vi "nism.step.p.fxp(modified).vi"(6 "calls per sample":u16, 7 "reset":bool, 8 "minimum pulse":u16, 11 "position setpoint":fxp<+/-,64,32>) -> (0 "position setpoint":fxp<+/-,64,32> format="%.42g", 1 "steps generated":i32, 2 "step":bool, 3 "direction":bool)   [LabVIEW 2015]
doc: "Generates the step and direction pulses necessary to perform stepper motor movement based on position setpoints."
uses:
  <vilib>/rvi/FXPMathLib/FxpDiv/subVIs/nifxpmath_Div_SimConfig.ctl
  <vilib>/rvi/FXPMathLib/FxpDiv/simVIs/DllFxpDivTemp_sub.vi
  <vilib>/rvi/FXPMathLib/FxpAdd/XNode/nifxpmath_Add.xnode
  <vilib>/rvi/FXPMathLib/FxpDiv/XNode/nifxpmath_Div.xnode
  <vilib>/rvi/FXPMathLib/FxpSub/XNode/nifxpmath_Sub.xnode
  <vilib>/Motion/MotorControl/NI_SoftMotion_MotorControlIP.lvlib
  <vilib>/rvi/FXPMathLib/sim/FxpSim.dll
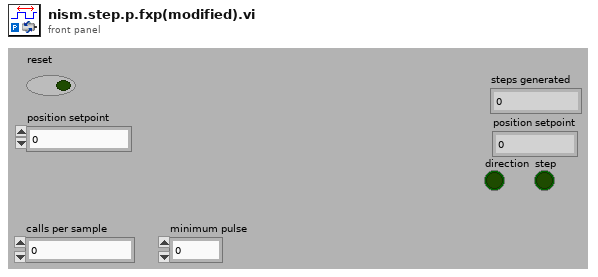
[diagram p1: front panel]
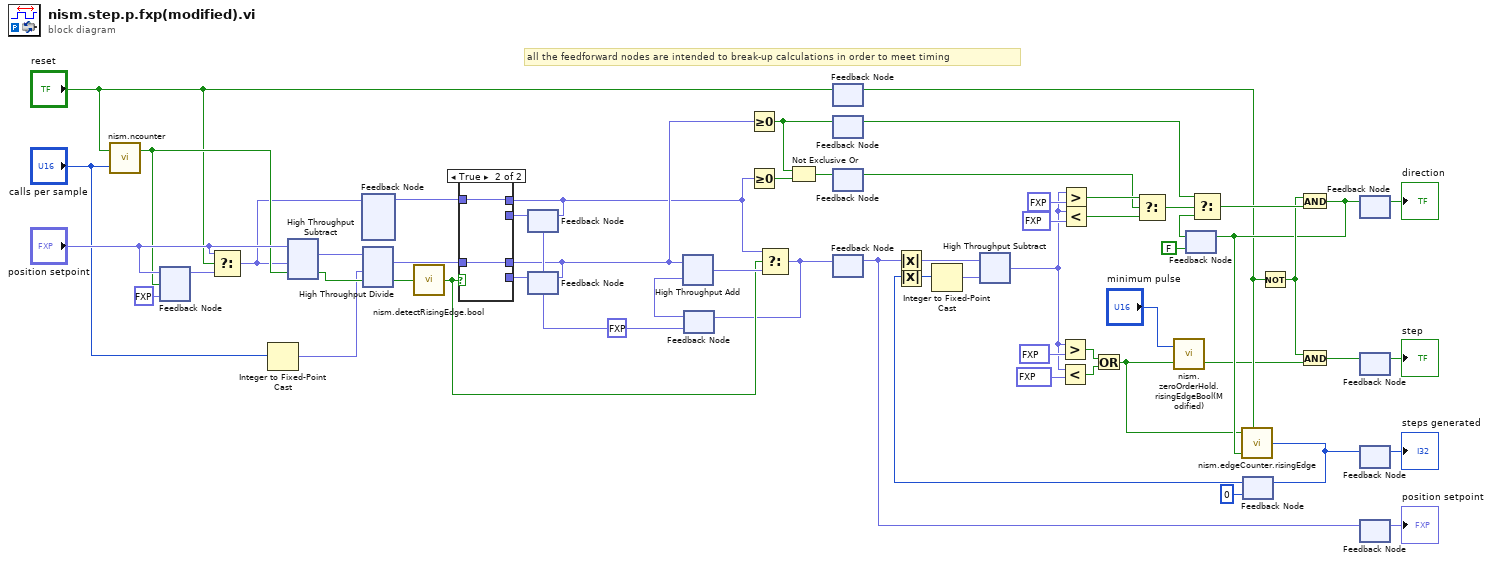
[diagram p0: block diagram]
diagram:
  w50 = fxp<+/-,48,16> 0.0 ("x+y")
  # "all the feedforward nodes are intended to break-up calculations in order to meet timing"
  n1 = call <vilib>:"nism.ncounter.vi"("n"="calls per sample", "reset"="reset") -> ("wrap"=w42:bool)  [unwired: 1 out]
  n2 = feedback #1(fxp<+/-,64,32> 0.0 ("x+y")) -> (w35:fxp<+/-,64,32>)
  n3 = feedback-in #1("position setpoint", w42) -> ()
  n4 = Select(t="position setpoint", s="reset", f=w35) -> (s? t:f=w33:fxp<+/-,64,32>)
  n5 = Integer to Fixed-Point Cast(integer="calls per sample") -> (fixed-point=w23:fxp<+,16,16>)  [unwired: 1 in]
  n6 = xnode ("High Throughput Subtract")("x"="position setpoint", "y"=w33, "input valid"=w42) -> ("x-y"=w28:fxp<+/-,32,16>, "output valid"=w27:bool)  [unwired: 1 in, 1 out]
  n7 = feedback #2() -> (w53:fxp<+/-,64,32>)  [unwired: 1 in]
  n8 = feedback-in #2(w33) -> ()
  n9 = xnode ("High Throughput Divide")("x"=w28, "y"=w23, "input valid"=w27) -> ("x/y"=w25:fxp<+/-,48,16>, "output valid"=w26:bool)  [unwired: 1 in, 1 out]
  n10 = call <vilib>:"nism.detectRisingEdge.bool.vi"("x"=w26) -> ("y"=w19:bool)
  n11 = feedback #3(w50) -> (w52:fxp<+/-,64,32>)
  n12 = feedback #4(w50) -> (w51:fxp<+/-,48,16>)
  n13 = case shown="True" w19 {
    tunnel: w53 -> [_ w62]
    tunnel: w25 -> [_ w61]
    tunnel: [w60 w62] -> w20
    tunnel: [w59 w61] -> w21
    tunnel: w52 -> [w60 _]
    tunnel: w51 -> [w59 _]
    frame False {
    }
    frame True {
    }
  }
  n14 = feedback-in #3(w20) -> ()
  n15 = feedback-in #4(w21) -> ()
  n16 = feedback #5(w50) -> (w55:fxp<+/-,64,32>)
  n17 = xnode ("High Throughput Add")("x"=w21, "y"=w55) -> ("x+y"=w49:fxp<+/-,64,32>)
  n18 = Greater Or Equal To 0?(x=w21) -> (x >= 0?=w9:bool)
  n19 = Greater Or Equal To 0?(x=w20) -> (x >= 0?=w29:bool)
  n20 = Select(t=w20, s=w19, f=w49) -> (s? t:f=w12:fxp<+/-,64,32>)
  n21 = feedback-in #5(w12) -> ()
  n22 = Not Exclusive Or(1:w29, 2:w9) -> (0:w11:bool)
  n23 = feedback #6() -> (w6:bool)  [unwired: 1 in]
  n24 = feedback-in #6("reset") -> ()
  n25 = feedback #7() -> (w8:bool)  [unwired: 1 in]
  n26 = feedback-in #7(w9) -> ()
  n27 = feedback #8() -> (w10:bool)  [unwired: 1 in]
  n28 = feedback-in #8(w11) -> ()
  n29 = feedback #9() -> (w5:fxp<+/-,64,32>)  [unwired: 1 in]
  n30 = feedback-in #9(w12) -> ()
  n31 = Absolute Value(x=w5) -> (abs(x)=w22:fxp<+,64,32>)
  n32 = feedback #10(FALSE) -> (w58:bool)
  n33 = feedback #11(0 ("rising edges")) -> (w32:i32)
  n34 = Absolute Value(x=w32) -> (abs(x)=w43:i32)
  n35 = Integer to Fixed-Point Cast(integer=w43) -> (fixed-point=w44:fxp<+/-,32,32>)  [unwired: 1 in]
  n36 = xnode ("High Throughput Subtract")("x"=w22, "y"=w44) -> ("x-y"=w39:fxp<+/-,32,1>)
  n37 = Greater?(x=w39, y=fxp<+/-,32,1> 0.75) -> (0:w36:bool)
  n38 = Less?(x=w39, y=fxp<+/-,32,1> -0.75) -> (x < y?=w37:bool)
  n39 = Greater?(x=w39, y=fxp<+/-,32,1> 0.5) -> (0:w46:bool)
  n40 = Less?(x=w39, y=fxp<+/-,32,1> -0.5) -> (x < y?=w45:bool)
  n41 = Or(x=w36, y=w37) -> (x .or. y?=w3:bool)
  n42 = Select(t=w46, s=w10, f=w45) -> (s? t:f=w41:bool)
  n43 = call "nism.zeroOrderHold.risingEdgeBool(Modified).vi"("min pulse"="minimum pulse", "input"=w3) -> ("output"=w2:bool)
  n44 = Select(t=w8, s=w41, f=w58) -> (s? t:f=w56:bool)
  n45 = Not(x=w6) -> (.not. x?=w30:bool)
  n46 = And(x=w30, y=w56) -> (x .and. y?=w17:bool)
  n47 = feedback-in #10(w17) -> ()
  n48 = call <vilib>:"nism.edgeCounter.risingEdge.vi"("input"=w3, "reset"=w6, "direction"=w17) -> ("rising edges"=w14:i32)  [unwired: 2 in]
  n49 = feedback-in #11(w14) -> ()
  n50 = And(x=w30, y=w2) -> (x .and. y?=w16:bool)
  n51 = feedback-in #12(w17) -> ()
  n52 = feedback #12() -> (→"direction":bool)  [unwired: 1 in]
  n53 = feedback #13() -> (→"step":bool)  [unwired: 1 in]
  n54 = feedback-in #13(w16) -> ()
  n55 = feedback #14() -> (→"steps generated":i32)  [unwired: 1 in]
  n56 = feedback-in #14(w14) -> ()
  n57 = feedback #15() -> (→"position setpoint":fxp<+/-,64,32>)  [unwired: 1 in]
  n58 = feedback-in #15(w5) -> ()
